vi "Load All Subitems.vi"(8 "error in (no error)":errorcluster, 11 "Application Data in":T1) -> (0 "error out":errorcluster, 3 "Application Data out":T1)   [LabVIEW 2017, in "DSF Configuration Utility.lvlib"]
uses:
  DSF Configuration Utility.lvlib
  Main VI/Application Data.ctl
  DSF Configuration API/1.0.0/Public/Controls/DSF Config Data RefNum.ctl
  Main VI/View Mode.ctl
  DSF Configuration API/1.0.0/Public/Read All Item IDs/Read All Plugin IDs.vi
  DSF Configuration API/1.0.0/DSF Configuration API.lvlib
panel:
  # "App\nData"
  # "App\nData"
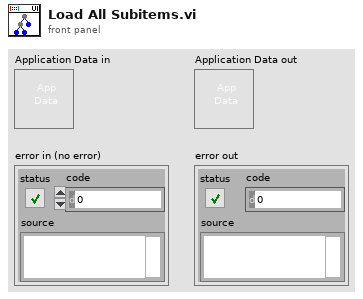
[diagram p1: front panel]
types:
  T1 = typedef "DSF Configuration Utility.lvlib/Application Data.ctl" = cluster{"Item Tree Control":refnum<vi>, "Value Tree Control":refnum<vi>, "DSF Refnum":T2, "Top-Level VI":refnum<vi>, "View State":T3, "menu reference":refnum<k9>}
  T2 = typedef "DSF Configuration API.lvlib/DSF Config Data RefNum.ctl" = refnum<k1>
  T3 = typedef "DSF Configuration Utility.lvlib/View Mode.ctl" = enum16{"Tree", "List"}
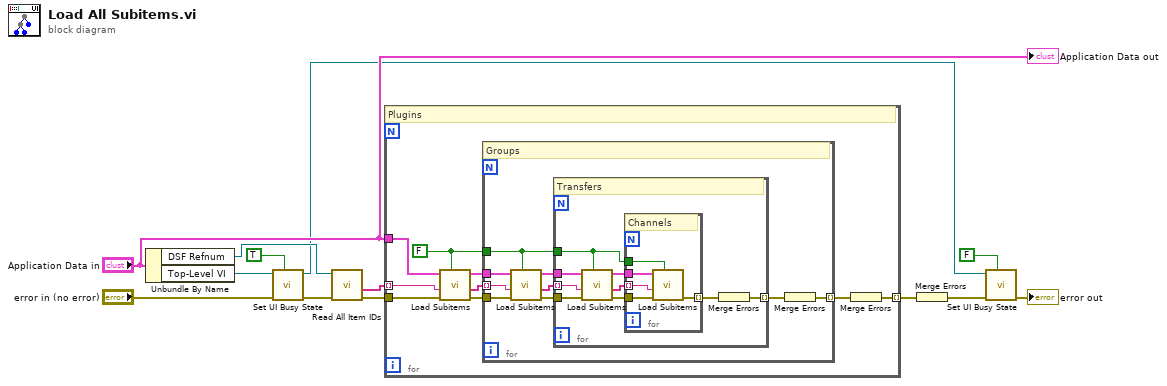
[diagram p0: block diagram]
diagram:
  n1 = Unbundle By Name("Application Data in") -> ("DSF Refnum"=w13:T2, "Top-Level VI"=w5:refnum<vi>)
  n2 = call "Set UI Busy State.vi"("Defer Panel Updates"=TRUE, "error in (no error)"="error in (no error)", "VI in"=w5) -> ("error out"=w6:errorcluster, "VI out"=w4:refnum<vi>)  [unwired: 7 in]
  n3 = call-poly "Read All Item IDs.vi"("error in (no error)"=w6, "dsf refnum"=w13) -> ("error out"=w9:errorcluster, "Plugin IDs"=w11:string[])  [unwired: 7 in, 1 out]
  n4 = for {
    tunnel: "Application Data in" -> [w22]
    tunnel: w11 -> [w21] mode=indexing
    tunnel: w9 -> [w18]
    tunnel: [w15] -> w8 mode=indexing
    w14 = FALSE ("defer fp updates?(T)")
    # "Plugins"
    n5 = call "Load Subitems.vi"("defer fp updates?(T)"=w14, "error in (no error)"=w18, "Tag"=w21, "Application Data in"=w22) -> ("error out"=w17:errorcluster, "item children"=w20:string[], "Application Data out"=w19:T1)  [unwired: 5 in]
    n6 = for {
      tunnel: w19 -> [w31]
      tunnel: w20 -> [w30] mode=indexing
      tunnel: w17 -> [w27]
      tunnel: [w24] -> w16 mode=indexing
      tunnel: w14 -> [w23]
      # "Groups"
      n7 = call "Load Subitems.vi"("defer fp updates?(T)"=w23, "error in (no error)"=w27, "Tag"=w30, "Application Data in"=w31) -> ("error out"=w26:errorcluster, "item children"=w28:string[], "Application Data out"=w29:T1)  [unwired: 5 in]
      n8 = for {
        tunnel: w29 -> [w40]
        tunnel: w28 -> [w37] mode=indexing
        tunnel: w26 -> [w36]
        tunnel: [w33] -> w25 mode=indexing
        tunnel: w23 -> [w32]
        # "Transfers"
        n9 = call "Load Subitems.vi"("defer fp updates?(T)"=w32, "error in (no error)"=w36, "Tag"=w37, "Application Data in"=w40) -> ("error out"=w35:errorcluster, "item children"=w39:string[], "Application Data out"=w38:T1)  [unwired: 5 in]
        n10 = for {
          tunnel: w38 -> [w45]
          tunnel: w39 -> [w44] mode=indexing
          tunnel: w35 -> [w43]
          tunnel: [w42] -> w34 mode=indexing
          tunnel: w32 -> [w41]
          # "Channels"
          n11 = call "Load Subitems.vi"("defer fp updates?(T)"=w41, "error in (no error)"=w43, "Tag"=w44, "Application Data in"=w45) -> ("error out"=w42:errorcluster)  [unwired: 5 in, 2 out]
        }
        n12 = Merge Errors(w34) -> (w33:errorcluster)
      }
      n13 = Merge Errors(w25) -> (w24:errorcluster)
    }
    n14 = Merge Errors(w16) -> (w15:errorcluster)
  }
  n15 = Merge Errors(w8) -> (w7:errorcluster)
  n16 = call "Set UI Busy State.vi"("Defer Panel Updates"=FALSE, "error in (no error)"=w7, "VI in"=w4) -> ("error out"=→"error out":errorcluster)  [unwired: 7 in, 1 out]
  "Application Data out" <- "Application Data in"
